vi "create_SMGR02.vi"(4 "error out in":errorcluster, 5 "array":waveform(i16)[][](array[waveform]), 6 "meas_point":i32, 7 "sync":waveform(i16)) -> (0 "error out":errorcluster, 3 "path":path)   [LabVIEW 2010]
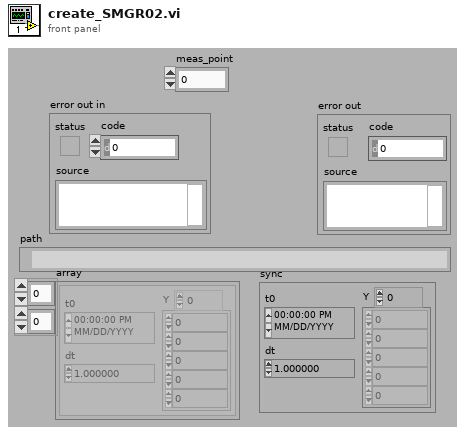
[diagram p1: front panel]
types:
  T1 = enum16{"open", "replace", "create", "open or create", "replace or create", "replace or create with confirmation"}
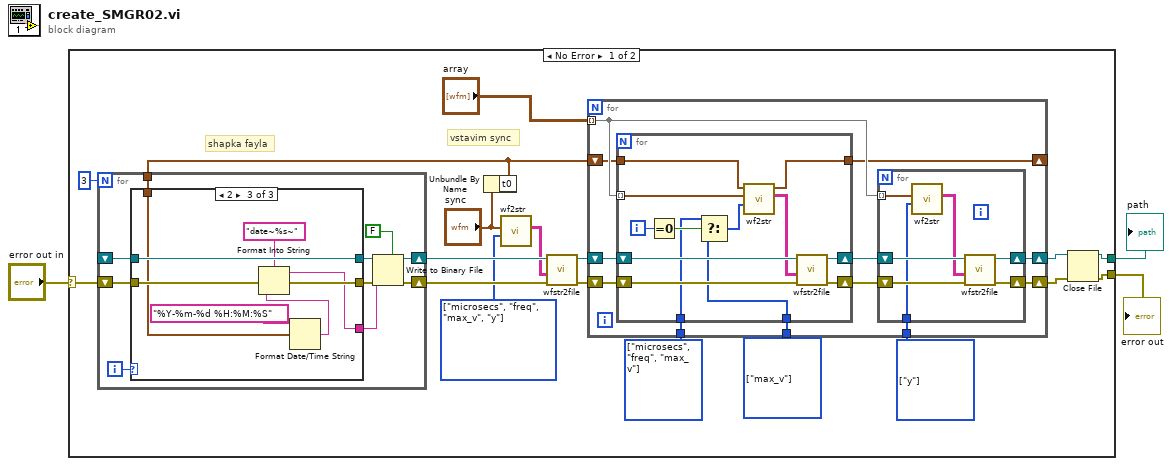
[diagram p0: block diagram]
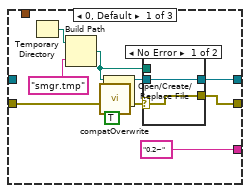
[diagram p2: hidden frame]
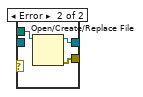
[diagram p3: hidden frame]
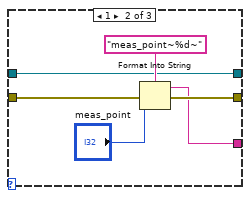
[diagram p4: hidden frame]
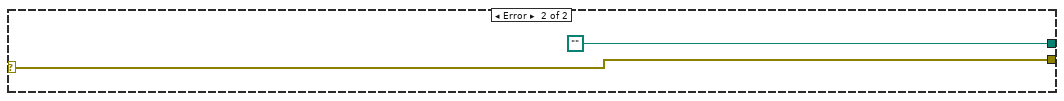
[diagram p5: hidden frame]
diagram:
  n1 = case shown="No Error" "error out in" {
    selector: "error out in" -> [w18 w95]
    tunnel: [w21 w95] -> w2
    tunnel: [w20 path ""] -> w1
    frame No Error {
      w11 = enum16{"microsecs", "freq", "max_v", "y"}[] [enum."y"] items=["microsecs", "freq", "max_v", "y"] ("fields")
      w12 = enum16{"microsecs", "freq", "max_v", "y"}[] [enum."max_v"] items=["microsecs", "freq", "max_v", "y"] ("fields")
      w13 = enum16{"microsecs", "freq", "max_v", "y"}[] [enum."microsecs", enum."freq", enum."max_v"] items=["microsecs", "freq", "max_v", "y"] ("fields")
      w14 = enum16{"microsecs", "freq", "max_v", "y"}[] [enum."microsecs", enum."freq", enum."max_v", enum."y"] items=["microsecs", "freq", "max_v", "y"] ("fields")
      # "vstavim sync"
      # "shapka fayla"
      n2 = Unbundle By Name("sync") -> ("t0"=w4:timestamp)
      n3 = for {
        N: 3 -> [_]
        shift-right: [w26] -> w16
        shift-left: _ -> [w29]
        shift-right: [w25] -> w17
        shift-left: w18 -> [w30]
        tunnel: w4 -> [w23]
        i -> [w31]
        n4 = case shown="2" w31 {
          tunnel: [w34 w49 w58] -> w28
          tunnel: [w35 w50 w60] -> w27
          tunnel: w30 -> [w36 w51 w59]
          tunnel: w29 -> [_ w50 w60]
          tunnel: ["0.2~" w48 w55] -> w24
          tunnel: w23 -> [_ _ w54]
          frame 0, Default {
            n5 = Temporary Directory() -> (w39:path)
            n6 = Build Path(base path=w39, name or relative path="smgr.tmp") -> (appended path=w37:path)
            n7 = call <vilib>:"compatOverwrite.vi"("overwrite (F)"=TRUE) -> ("overwrite?"=w32:T1)
            n8 = Open/Create/Replace File(file path (use dialog)=w37, error in=w36, operation (0:open)=w32) -> (refnum out=w42:refnum<file>, error out=w41:errorcluster)  [unwired: 3 in, 1 out]
            n9 = case shown="No Error" w41 {
              selector: w41 -> [w44 _]
              tunnel: [w44 w46] -> w34
              tunnel: w42 -> [w43 _]
              tunnel: [w43 w45] -> w35
              tunnel: w37 -> [_ w47]
              frame No Error {
              }
              frame Error {
                n10 = Open/Create/Replace File(file path (use dialog)=w47) -> (refnum out=w45:refnum<file>, error out=w46:errorcluster)  [unwired: 5 in, 1 out]
              }
            }
          }
          frame 1 {
            n11 = Format Into String(format string="meas_point~%d~", error in=w51, "meas_point") -> (resulting string=w48:string, error out=w49:errorcluster)  [unwired: 1 in]
          }
          frame 2 {
            n12 = Format Date/Time String(time format string (%c)="%Y-%m-%d %H:%M:%S", seconds (now)=w54) -> (date/time string=w57:string)  [unwired: 1 in]
            n13 = Format Into String(format string="date~%s~", error in=w59, w57) -> (resulting string=w55:string, error out=w58:errorcluster)  [unwired: 1 in]
          }
        }
        n14 = Write to Binary File(file (use dialog)=w27, data=w24, error in=w28, 5:FALSE ("prepend array or string size? (T)")) -> (refnum out=w26:refnum<file>, error out=w25:errorcluster)  [unwired: 2 in, 1 out]
      }
      n15 = call "wf2str.vi"("fields"=w14, "Signal"="sync") -> ("Table"=w15:string[][])  [unwired: 3 in, 2 out]
      n16 = call "wfstr2file.vi"("error in"=w17, "Array"=w15, "Byte Stream File Refnum"=w16) -> ("error out"=w9:errorcluster, "Byte Stream File Refnum 2"=w10:refnum<file>)  [unwired: 3 in]
      n17 = for {
        tunnel: "array" -> [w71] mode=indexing
        shift-right: [w65] -> w8
        shift-left: w10 -> [w67]
        shift-right: [w64] -> w7
        shift-left: w9 -> [w66]
        tunnel: w13 -> [w73]
        tunnel: w12 -> [w72]
        tunnel: w11 -> [w70]
        shift-right: [w62] -> _
        shift-left: w4 -> [w63]
        n18 = for {
          tunnel: w71 -> [w83] mode=indexing
          shift-right: [w93] -> w69
          shift-left: w67 -> [w90]
          shift-right: [w92] -> w68
          shift-left: w66 -> [w91]
          tunnel: w73 -> [w86]
          tunnel: w72 -> [w85]
          tunnel: w63 -> [w82]
          tunnel: [w81] -> w62
          i -> [w87]
          n19 = Equal To 0?(x=w87) -> (x = 0?=w88:bool)
          n20 = Select(t=w86, s=w88, f=w85) -> (s? t:f=w84:enum16{"microsecs", "freq", "max_v", "y"}[])
          n21 = call "wf2str.vi"("fields"=w84, "Signal"=w83, "PrevTime"=w82) -> ("Table"=w89:string[][], "NextTime"=w81:timestamp)  [unwired: 2 in, 1 out]
          n22 = call "wfstr2file.vi"("error in"=w91, "Array"=w89, "Byte Stream File Refnum"=w90) -> ("error out"=w92:errorcluster, "Byte Stream File Refnum 2"=w93:refnum<file>)  [unwired: 3 in]
        }
        n23 = for {
          tunnel: w71 -> [w75] mode=indexing
          shift-right: [w80] -> w65
          shift-left: w69 -> [w77]
          shift-right: [w79] -> w64
          shift-left: w68 -> [w78]
          tunnel: w70 -> [w74]
          n24 = call "wf2str.vi"("fields"=w74, "Signal"=w75) -> ("Table"=w76:string[][])  [unwired: 3 in, 2 out]
          n25 = call "wfstr2file.vi"("error in"=w78, "Array"=w76, "Byte Stream File Refnum"=w77) -> ("error out"=w79:errorcluster, "Byte Stream File Refnum 2"=w80:refnum<file>)  [unwired: 3 in]
        }
      }
      n26 = Close File(refnum=w8, error in=w7) -> (path=w20:path, error out=w21:errorcluster)
    }
    frame Error {
    }
  }
  "error out" <- w2
  "path" <- w1
